vi "Drive Main.vi"(0 "spin":dbl, 1 "In x":dbl, 2 "In y":dbl) -> ()   [LabVIEW 2023]
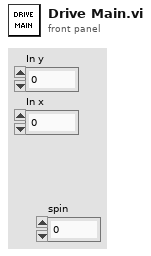
[diagram p1: front panel]
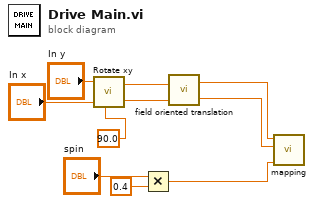
[diagram p0: block diagram]
diagram:
  n1 = call "Rotate xy.vi"("In y"="In y", "In x"="In x", "Rotate degrees"=90.0) -> ("Out y"=w6:dbl, "Out x"=w5:dbl)  [unwired: 2 in]
  n2 = Multiply(x="spin", y=0.4) -> (x*y=w7:dbl)
  n3 = call "field oriented translation.vi"("x in"=w5, "y in"=w6) -> ("x out"=w9:dbl, "y out"=w10:dbl)
  n4 = call "mapping.vi"("spin"=w7, "x"=w9, "y"=w10) -> ()  [unwired: 9 in]
